vi "IPS120_to_DSC.vi"(0 "str":string[](array[string])=["CLMP"], 1 "str var":refnum<k21>[](array[refnum])=["ni.var.psp://housesoftheholy/DR200/DR200_Magnet_Status_Activity", "ni.var.psp://housesoftheholy/DR200/DR200_Magnet_Status_Mode", "ni.var.psp://housesoftheholy/DR200/DR200_Magnet_Status_Switch_Heater", "ni.var.psp://housesoftheholy/DR200/DR200_Magnet_Status_System"], 2 "dbl":dbl[](array[numeric])=[0.0, -0.0, 0.0, 0.91, -0.0002, -0.0003, 81.9328, 94.8099], 3 "dbl var":refnum<k21>[](array[refnum])=["ni.var.psp://housesoftheholy/DR200/DR200_Magnet_Field", "ni.var.psp://housesoftheholy/DR200/DR200_Magnet_Field_Target", "ni.var.psp://housesoftheholy/DR200/DR200_Magnet_PS_Current", "ni.var.psp://housesoftheholy/DR200/DR200_Magnet_PS_Field", "ni.var.psp://housesoftheholy/DR200/DR200_Magnet_PS_Voltage", "ni.var.psp://housesoftheholy/DR200/DR200_Magnet_Rate_Target"]) -> ()   [LabVIEW 2016, in "IPS-120.lvlib"]
uses:
  IPS-120.lvlib
panel:
  # "DR200 IPS120 to DSC"
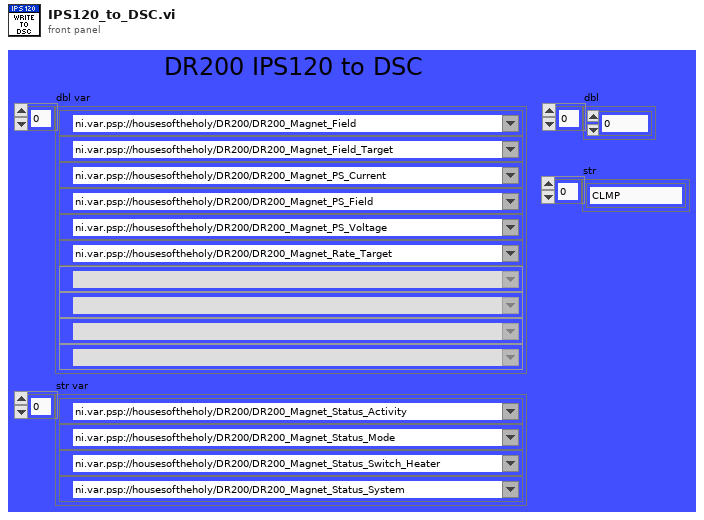
[diagram p1: front panel]
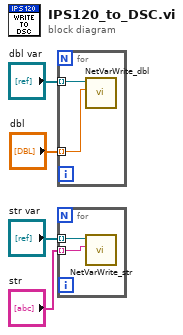
[diagram p0: block diagram]
diagram:
  n1 = for {
    tunnel: "dbl var" -> [w6] mode=indexing
    tunnel: "dbl" -> [w5] mode=indexing
    n2 = call "NetVarWrite_dbl.vi"("Numeric"=w5, "Refnum in"=w6) -> ()  [unwired: 10 in]
  }
  n3 = for {
    tunnel: "str var" -> [w8] mode=indexing
    tunnel: "str" -> [w7] mode=indexing
    n4 = call "NetVarWrite_str.vi"("String"=w7, "Refnum in"=w8) -> ()  [unwired: 10 in]
  }
